vi "about_launcher_v1.0.vi"(8 "error in (no error)":errorcluster) -> (0 "error out":errorcluster)   [LabVIEW 2025]
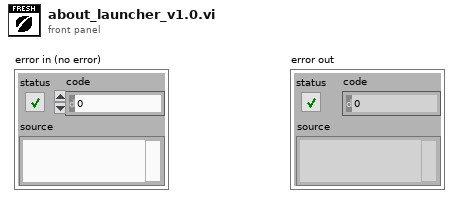
[diagram p1: front panel]
types:
  T1 = enum32{"Invalid", "Standard", "Closed", "Hidden", "Minimized", "Maximized"}
  T2 = enum32{"Bad", "Idle", "Run top level", "Running"}
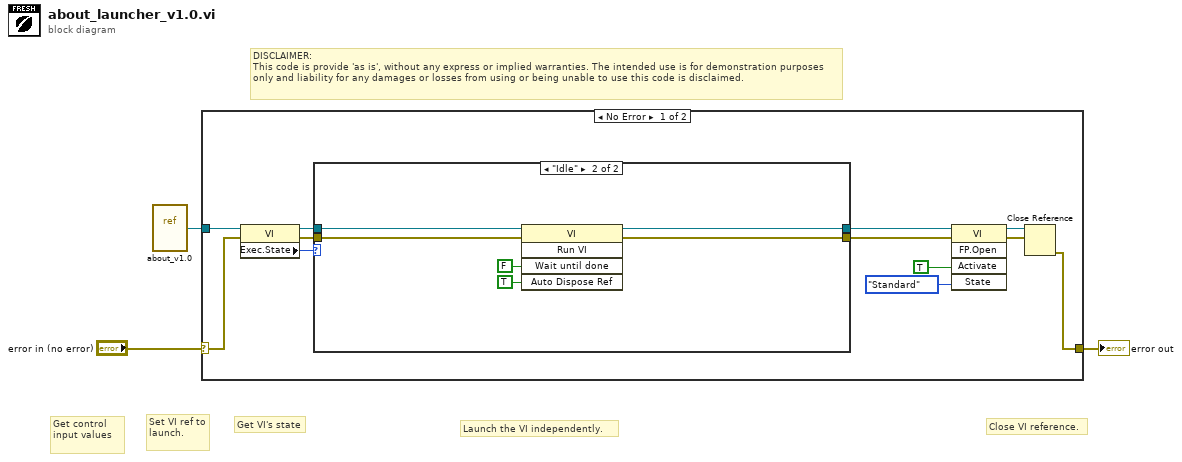
[diagram p0: block diagram]
diagram:
  # "Close VI reference."
  # "Launch the VI independently."
  # "Get VI's state"
  # "Set VI ref to launch."
  # "Get control input values"
  # "DISCLAIMER:\nThis code is provide 'as is', without any express or implied warranties. The intended use is for demonstration purposes only and liability for any damages or losses from using or being unable to use this code is disclaimed."
  n1 = vi-ref "about_v1.0.vi"() -> (w3:refnum<vi>)
  n2 = case shown="No Error" "error in (no error)" {
    selector: "error in (no error)" -> [w4 w24]
    tunnel: w3 -> [w11 _]
    tunnel: [w12 w24] -> w1
    frame No Error {
      n3 = property class="VI"(reference=w11, error in=w4) -> (reference out=w14:refnum<vi>, error out=w13:errorcluster, "Exec.State"=w15:T2)
      n4 = case shown="\"Idle\"" w15 {
        tunnel: w14 -> [w16 w19]
        tunnel: w13 -> [w17 w18]
        tunnel: [w16 w21] -> w8
        tunnel: [w17 w20] -> w5
        frame Default {
        }
        frame "Idle" {
          n5 = invoke class="VI" method="Run VI"(reference=w19, error in=w18, "Wait until done"=FALSE ("Wait Until Done"), "Auto Dispose Ref"=TRUE ("Auto Dispose Reference")) -> (reference out=w21:refnum<vi>, error out=w20:errorcluster)  [unwired: 1 in, 3 out]
        }
      }
      n6 = invoke class="VI" method="FP.Open"(reference=w8, error in=w5, "Activate"=TRUE ("Activate?"), "State"=T1."Standard") -> (reference out=w7:refnum<vi>, error out=w6:errorcluster)  [unwired: 1 in, 3 out]
      n7 = Close Reference(reference=w7, error in (no error)=w6) -> (error out=w12:errorcluster)
    }
    frame Error {
    }
  }
  "error out" <- w1
